vi "AVS_GetLambda.vi"(0 "a_hDevice":i32, 11 "a_pWaveLength":dbl[](array[numeric])) -> (4 "Output Value":i32, 15 "a_pWaveLength":dbl[](array[numeric]))   [LabVIEW 2016]
uses:
  libavs.so
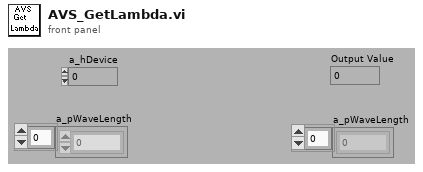
[diagram p1: front panel]
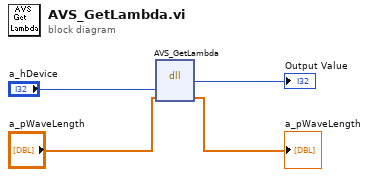
[diagram p0: block diagram]
diagram:
  n1 = dll-call lib="home/harini/tcs/ts_sedspectrometer/ss_sedspectrometer/VIs/libavs.so" fn="AVS_GetLambda"("a_hDevice"="a_hDevice", "a_pWaveLength"="a_pWaveLength") -> ("return type"=→"Output Value":i32, "a_pWaveLength"=→"a_pWaveLength":dbl[])  [unwired: 4 in, 2 out]
